vi "Transmit.vi"(8 "error in":errorcluster, 11 "framework in":refnum<class "Framework.lvclass">) -> (0 "error out":errorcluster, 3 "framework out":refnum<class "Framework.lvclass">)   [LabVIEW 2019, in "DSF Core.lvlib" / "Framework.lvclass"]
uses:
  Framework.lvclass
  Framework States.ctl
  Framework.lvclass/Framework.ctl
  Performance/Performance.lvclass/Performance.ctl
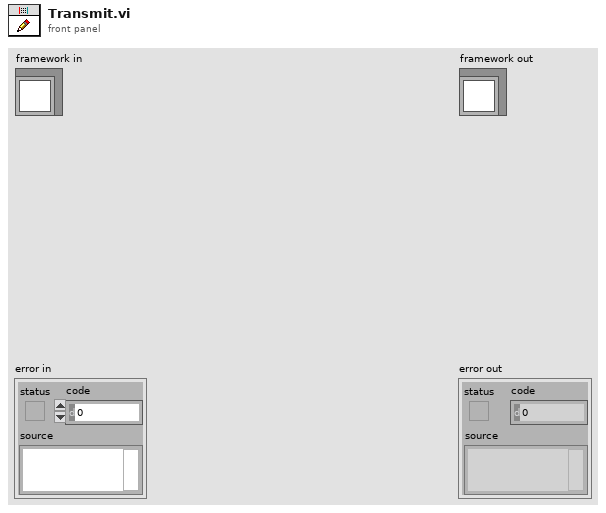
[diagram p1: front panel]
types:
  T1 = typedef "DSF Core.lvlib/Framework.lvclass/Framework States.ctl" = enum8{"Uninitialized", "Initialized", "Start", "Rx", "Tx", "Shutdown"}
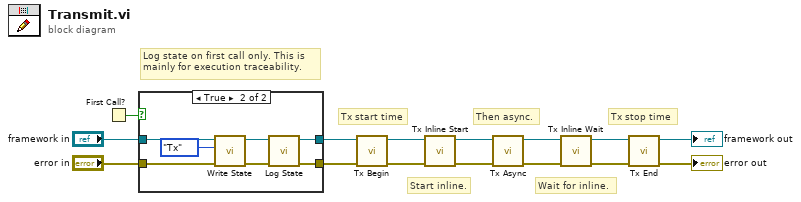
[diagram p0: block diagram]
diagram:
  # "Tx stop time"
  # "Tx start time"
  # "Log state on first call only. This is mainly for execution traceability."
  # "Wait for inline."
  # "Start inline."
  # "Then async."
  n1 = First Call?() -> (First Call?: T/F=w7:bool)
  n2 = case shown="True" w7 {
    tunnel: "error in" -> [w16 w21]
    tunnel: "framework in" -> [w17 w20]
    tunnel: [w16 w19] -> w10
    tunnel: [w17 w18] -> w11
    frame False {
    }
    frame True {
      n3 = call "Write State.vi"("error in (no error)"=w21, "state"=Framework_States."Tx", "Framework in"=w20) -> ("error out"=w22:errorcluster, "Framework out"=w23:refnum<class "Framework.lvclass">)  [unwired: 7 in]
      n4 = call "Log State.vi"("error in (no error)"=w22, "Framework in"=w23) -> ("error out"=w19:errorcluster, "Framework out"=w18:refnum<class "Framework.lvclass">)  [unwired: 8 in]
    }
  }
  n5 = call "Tx Begin.vi"("error in (no error)"=w10, "Framework in"=w11) -> ("error out"=w5:errorcluster, "Framework out"=w6:refnum<class "Framework.lvclass">)  [unwired: 8 in]
  n6 = call "Tx Inline Start.vi"("error in (no error)"=w5, "Framework in"=w6) -> ("error out"=w3:errorcluster, "Framework out"=w4:refnum<class "Framework.lvclass">)  [unwired: 8 in]
  n7 = call "Tx Async.vi"("error in (no error)"=w3, "Framework in"=w4) -> ("error out"=w1:errorcluster, "Framework out"=w2:refnum<class "Framework.lvclass">)  [unwired: 8 in]
  n8 = call "Tx Inline Wait.vi"("error in (no error)"=w1, "Framework in"=w2) -> ("error out"=w12:errorcluster, "Framework out"=w13:refnum<class "Framework.lvclass">)  [unwired: 8 in]
  n9 = call "Tx End.vi"("error in"=w12, "framework in"=w13) -> ("error out"=→"error out":errorcluster, "framework out"=→"framework out":refnum<class "Framework.lvclass">)  [unwired: 8 in]
